vi "Check Column.vi"(8 "error in (no error)":errorcluster, 11 "Composed Column in":refnum<class "Composed Column.lvclass">) -> (0 "error out":errorcluster, 3 "Composed Column out":refnum<class "Composed Column.lvclass">)   [LabVIEW 2020, in "Composed Columns.lvlib" / "Composed Column.lvclass"]
uses:
  Composed Column.lvclass
  Composed Column.lvclass/Composed Column.ctl
  Check Manager/Constraint Manager.lvclass
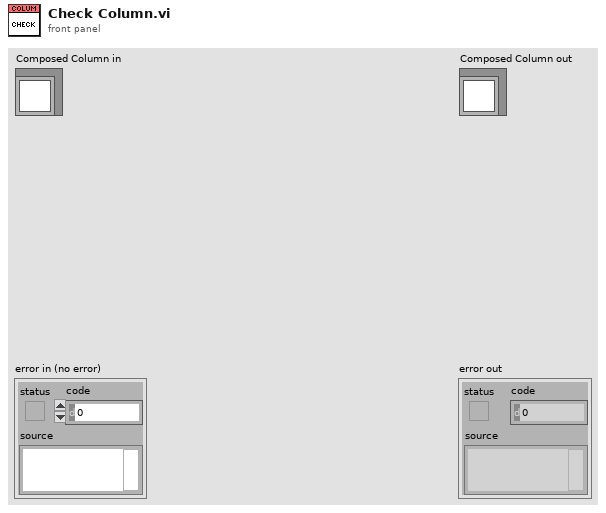
[diagram p1: front panel]
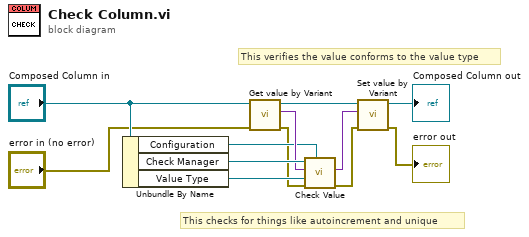
[diagram p0: block diagram]
diagram:
  # "This verifies the value conforms to the value type"
  # "This checks for things like autoincrement and unique"
  n1 = Unbundle By Name("Composed Column in") -> ("Configuration"=w8:refnum<class "Column Configuration.lvclass">, "Check Manager"=w12:refnum<class "Constraint Manager.lvclass">, "Value Type"=w7:refnum<class "Value Type.lvclass">)
  n2 = call-dynamic "Get value by Variant.vi"("error in (no error)"="error in (no error)", "Column in"="Composed Column in") -> ("error out"=w3:errorcluster, "Variant"=w11:variant, "Column out"=w10:refnum<class "Composed Column.lvclass">)  [unwired: 7 in]
  n3 = call-dynamic "Check Value.vi"("Column Configuration"=w8, "error in (no error)"=w3, "Value Type"=w7, "Value In"=w11, "Check Manager in"=w12) -> ("error out"=w2:errorcluster, "Value Out"=w9:variant)  [unwired: 4 in, 1 out]
  n4 = call-dynamic "Set value by Variant.vi"("error in (no error)"=w2, "Variant"=w9, "Column in"=w10) -> ("error out"=→"error out":errorcluster, "Column out"=→"Composed Column out":refnum<class "Composed Column.lvclass">)  [unwired: 7 in]
